vi "main.vi"() -> ()   [LabVIEW 2016]
uses:
  device/device.ctl
panel:
  out "Log":string
  in  "Temp":dbl
  in  "D":dbl=300.0
  in  "I":dbl=0.03
  in  "P":dbl=10.0
  in  "stop":bool
  in  "Device in":T1
  out "Waveform Chart":cluster{dbl, dbl, dbl, dbl}(graph)
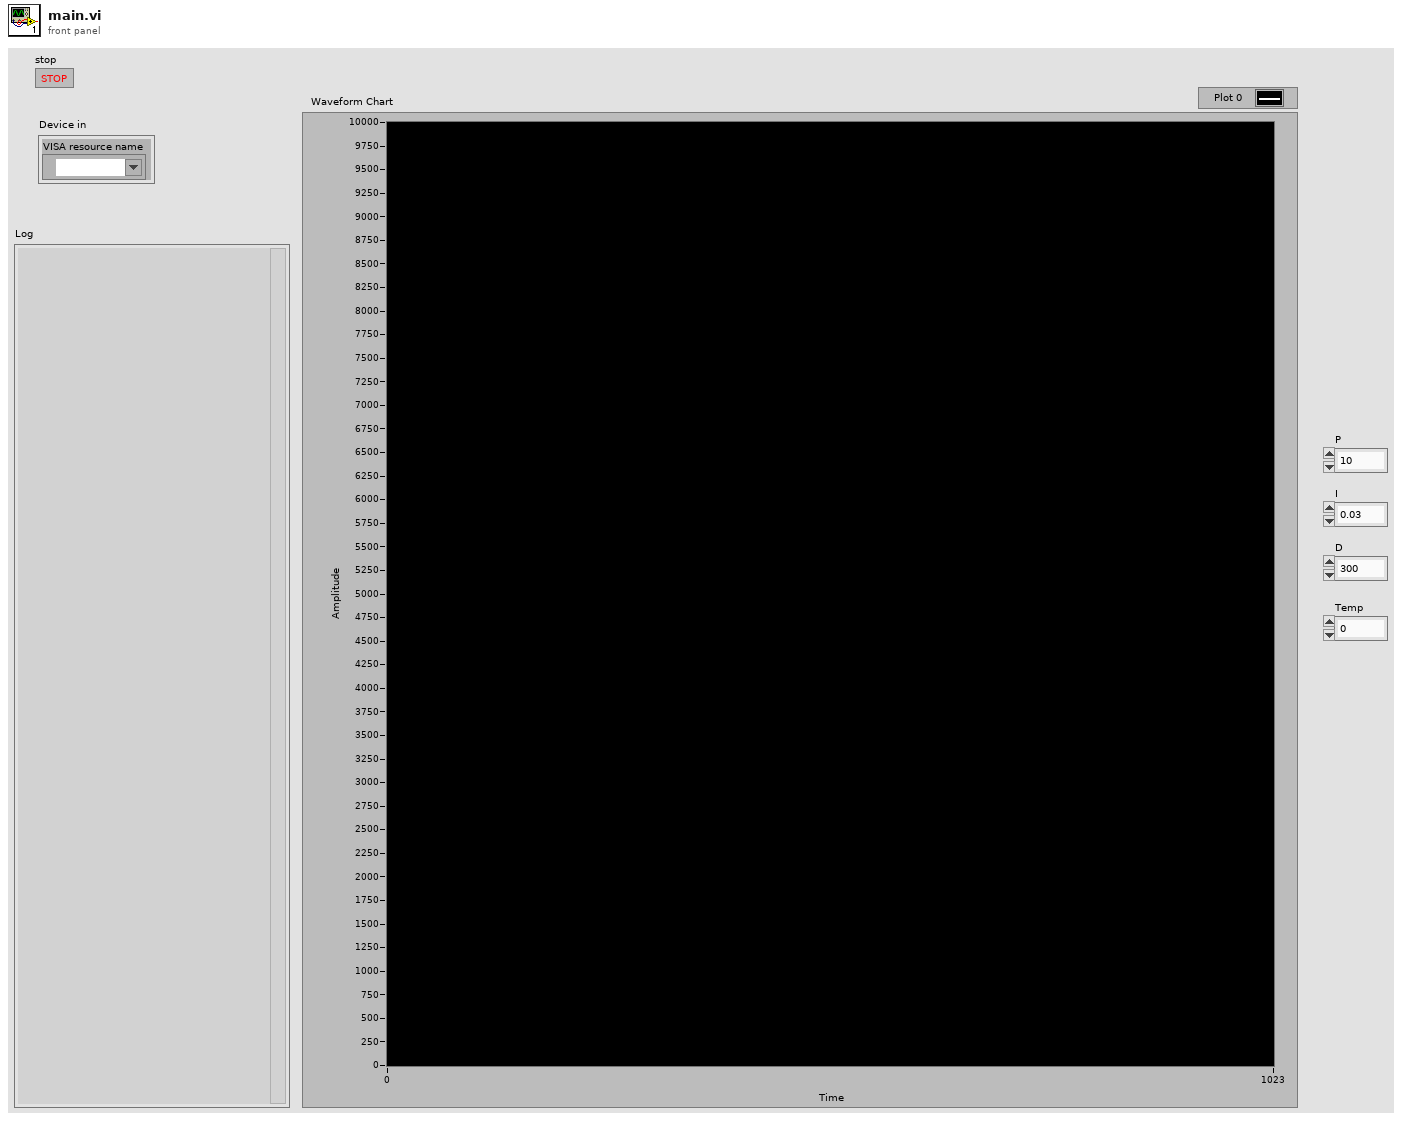
[diagram p1: front panel]
types:
  T1 = typedef "device.ctl" = cluster{"VISA resource name":refnum<visa-resource-name>}
  T2 = typedef "queues.ctl" = cluster{"Data received":refnum<queue>, "Data to transmit":refnum<queue>, "Error notifier":refnum<notifier>, "Tx semaphore":T3}
  T3 = typedef "Semaphore RefNum" = refnum<k1>
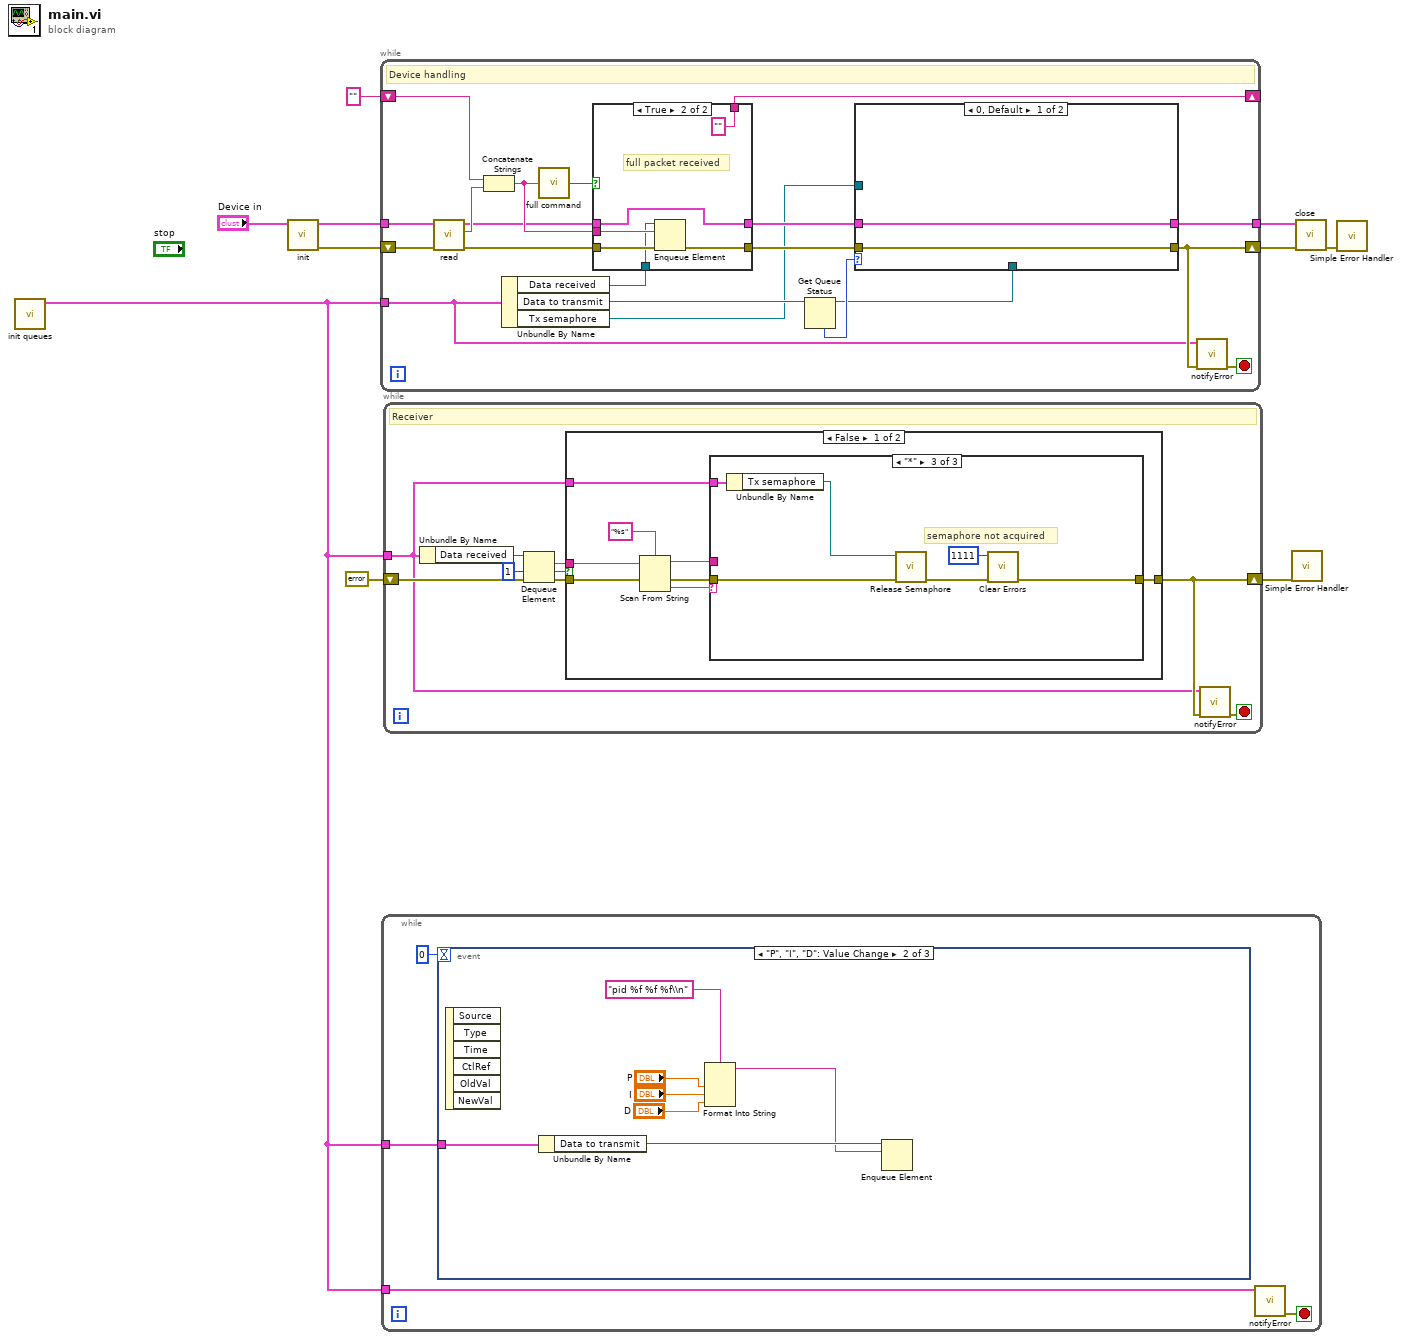
[diagram p0: block diagram]
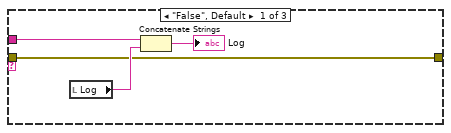
[diagram p2: hidden frame]
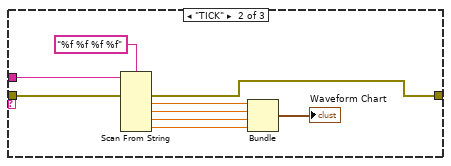
[diagram p3: hidden frame]
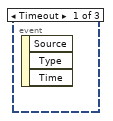
[diagram p5: hidden frame]
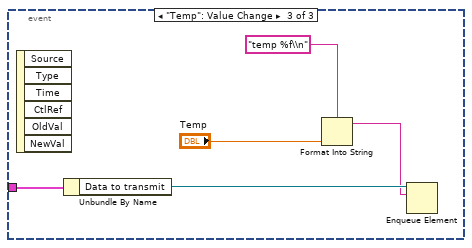
[diagram p6: hidden frame]
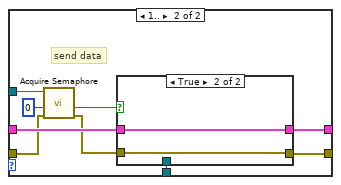
[diagram p7: hidden frame]
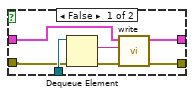
[diagram p8: hidden frame]
diagram:
  n1 = call "init queues.vi"() -> ("output device queues"=w3:T2)  [unwired: 10 in, 1 out]
  n2 = call "init.vi"("Device in"="Device in") -> ("error out"=w9:errorcluster, "Device out"=w5:T1)  [unwired: 9 in]
  n3 = while "Device handling" {
    tunnel: w5 -> [w20]
    shift-right: [w27] -> _
    shift-left: "" ("data") -> [w28]
    shift-right: [w14] -> w7
    shift-left: w9 -> [w30]
    tunnel: w3 -> [w13]
    tunnel: [w15] -> w6
    stop <- w12 stop-if-true
    # "Device handling"
    n4 = call "read.vi"("error in (no error)"=w30, "Device in"=w20) -> ("error out"=w21:errorcluster, "data"=w29:string, "Device out"=w16:T1)  [unwired: 7 in]
    n5 = Concatenate Strings(w28, w29) -> (w25:string)
    n6 = Unbundle By Name(w13) -> ("Data received"=w24:refnum<queue>, "Data to transmit"=w23:refnum<queue>, "Tx semaphore"=w11:T3)
    n7 = call "full command.vi"("Command string"=w25) -> ("Full command"=w26:bool)
    n8 = case shown="True" w26 {
      tunnel: w21 -> [w52 w57]
      tunnel: w25 -> [w53 w58]
      tunnel: [w53 ""] -> w27
      tunnel: [w52 w56] -> w19
      tunnel: w24 -> [_ w55]
      tunnel: [w51 w54] -> w17
      tunnel: w16 -> [w51 w54]
      frame False {
      }
      frame True {
        # "full packet received"
        n9 = Enqueue Element(queue=w55, element=w58, error in (no error)=w57) -> (error out=w56:errorcluster)  [unwired: 1 in, 2 out]
      }
    }
    n10 = Get Queue Status(queue=w23) -> (queue out=w18:refnum<queue>, # elements in queue=w22:i32)  [unwired: 2 in, 6 out]
    n11 = case shown="0, Default" w22 {
      tunnel: w18 -> [_ w41]
      tunnel: w19 -> [w31 w36]
      tunnel: w17 -> [w32 w40]
      tunnel: [w32 w39] -> w15
      tunnel: [w31 w33] -> w14
      tunnel: w11 -> [_ w37]
      frame 0, Default {
      }
      frame 1.. {
        # "send data"
        n12 = call <vilib>:"Acquire Semaphore.vi"("error in (no error)"=w36, "ms timeout (-1)"=0, "semaphore"=w37) -> ("error out"=w35:errorcluster, "timed out"=w34:bool)  [unwired: 2 in, 1 out]
        n13 = case shown="True" w34 {
          tunnel: w41 -> [w48 _]
          tunnel: w40 -> [w45 w49]
          tunnel: [w44 w49] -> w39
          tunnel: w35 -> [w43 w50]
          tunnel: [w42 w50] -> w33
          frame False {
            n14 = Dequeue Element(queue=w48, error in (no error)=w43) -> (element=w47:string, error out=w46:errorcluster)  [unwired: 1 in, 2 out]
            n15 = call "write.vi"("error in (no error)"=w46, "data"=w47, "Device in"=w45) -> ("error out"=w42:errorcluster, "Device out"=w44:T1)  [unwired: 7 in]
          }
          frame True {
          }
        }
      }
    }
    n16 = call "notifyError.vi"("error in (no error)"=w14, "data passing"=w13) -> ("error out"=w12:errorcluster)  [unwired: 8 in]
  }
  n17 = while {
    tunnel: w3 -> [w60]
    tunnel: w3 -> [w62]
    stop <- w61 stop-if-true
    n18 = event shown="[1] \"P\", \"I\", \"D\": Value Change" {
      selector: _ -> [_ _ _]
      dyn-events: _ -> [_ _ _]
      timeout: 0 -> [_ _ _]
      tunnel: w60 -> [_ w65 w73]
      event Timeout {
        n19 = event-data() -> ()  [unwired: 1 in, 3 out]
      }
      event "P", "I", "D": Value Change {
        n20 = event-data() -> ()  [unwired: 1 in, 6 out]
        n21 = Unbundle By Name(w65) -> ("Data to transmit"=w66:refnum<queue>)
        n22 = Format Into String(format string="pid %f %f %f\\n", "P", "I", "D") -> (resulting string=w64:string)  [unwired: 2 in, 1 out]
        n23 = Enqueue Element(queue=w66, element=w64) -> ()  [unwired: 2 in, 3 out]
      }
      event "Temp": Value Change {
        n24 = event-data() -> ()  [unwired: 1 in, 6 out]
        n25 = Unbundle By Name(w73) -> ("Data to transmit"=w72:refnum<queue>)
        n26 = Format Into String(format string="temp %f\\n", "Temp") -> (resulting string=w71:string)  [unwired: 2 in, 1 out]
        n27 = Enqueue Element(queue=w72, element=w71) -> ()  [unwired: 2 in, 3 out]
      }
    }
    n28 = call "notifyError.vi"("data passing"=w62) -> ("error out"=w61:errorcluster)  [unwired: 9 in]
  }
  n29 = while {
    tunnel: w3 -> [w76]
    shift-right: [w77] -> w2
    shift-left: errorcluster {"status"=FALSE, "code"=0, "source"=""} ("error in (no error)") -> [w83]
    stop <- w78 stop-if-true
    # "Receiver"
    n30 = Unbundle By Name(w76) -> ("Data received"=w84:refnum<queue>)
    n31 = Dequeue Element(queue=w84, timeout in ms (-1)=1, error in (no error)=w83) -> (element=w81:string, timed out?=w79:bool, error out=w80:errorcluster)  [unwired: 1 out]
    n32 = case shown="False" w79 {
      tunnel: w81 -> [w92 _]
      tunnel: w80 -> [w91 w112]
      tunnel: [w85 w112] -> w77
      tunnel: w76 -> [w87 _]
      frame False {
        n33 = Scan From String(format string="%s", input string=w92, error in=w91) -> (remaining string=w88:string, error out=w86:errorcluster, output 1=w89:string)  [unwired: 2 in, 1 out]
        n34 = case shown="\"*\"" w89 {
          tunnel: [w93 w102 w107] -> w85
          tunnel: w88 -> [w94 w98 _]
          tunnel: w87 -> [_ _ w111]
          tunnel: w86 -> [w93 w97 w109]
          frame "False", Default {
            n35 = local read "Log"() -> (w96:string)
            n36 = Concatenate Strings(w94, w96) -> (→"Log":string)
          }
          frame "TICK" {
            n37 = Scan From String(format string="%f %f %f %f", input string=w98, error in=w97) -> (error out=w102:errorcluster, output 1=w104:dbl, output 2=w103:dbl, output 3=w100:dbl, output 4=w99:dbl)  [unwired: 5 in, 2 out]
            n38 = Bundle(w104, w103, w100, w99) -> (→"Waveform Chart":cluster{dbl, dbl, dbl, dbl})  [unwired: 1 in]
          }
          frame "*" {
            # "semaphore not acquired"
            n39 = Unbundle By Name(w111) -> ("Tx semaphore"=w110:T3)
            n40 = call <vilib>:"Release Semaphore.vi"("error in (no error)"=w109, "semaphore"=w110) -> ("error out"=w108:errorcluster)  [unwired: 4 in, 1 out]
            n41 = call <vilib>:"Clear Errors.vi"("error in (no error)"=w108, "specific error code to clear (0: all)"=1111) -> ("error out"=w107:errorcluster)  [unwired: 4 in, 1 out]
          }
        }
      }
      frame True {
      }
    }
    n42 = call "notifyError.vi"("error in (no error)"=w77, "data passing"=w76) -> ("error out"=w78:errorcluster)  [unwired: 8 in]
  }
  n43 = call <vilib>:"Simple Error Handler.vi"("error in (no error)"=w2) -> ()  [unwired: 4 in, 5 out]
  n44 = call "close.vi"("error in (no error)"=w7, "Device in"=w6) -> ("error out"=w1:errorcluster)  [unwired: 8 in, 1 out]
  n45 = call <vilib>:"Simple Error Handler.vi"("error in (no error)"=w1) -> ()  [unwired: 4 in, 5 out]
